vi "Autonomous Independent.vi"() -> ()   [LabVIEW 2016]
doc: "This VI is called when autonomous begins, and will automatically be terminated when autonomous ends. You can carry out timed or sensor driven robot movement independently without needing to return to the caller."
uses:
  <vilib>/Rock Robotics/WPI/Solenoid/WPI_SolenoidValue.ctl
  <vilib>/Rock Robotics/WPI/Utilities/WPI_GetSetVariantRefNum.vi
  <vilib>/Rock Robotics/Network Tables/NT Read String.vi
  <vilib>/Rock Robotics/Network Tables/NT Write Numeric Array.vi
  <vilib>/Rock Robotics/WPI/RobotDrive/WPI_RobotDriveArcadeDrive_Standard(NoSaturation).vi
  <vilib>/Rock Robotics/WPI/Solenoid/WPI_SolenoidSetEnum.vi
panel:
  in  "Reset":bool
  out "Current Movement, for debugging":T1 {"Y Joystick Value" scale=1.0..-1.0; "X Joystick Value" scale=-1.0..1.0}
  in  "Array of robot movements":T2(array[cluster])=[{"X Joystick Value"=0.39393939393939403, "Y Joystick Value"=0.0, "Delay (sec)"=1.0, "Movement Name"="turn"}, {"X Joystick Value"=-0.3737373737373737, "Y Joystick Value"=0.0, "Delay (sec)"=1.0, "Movement Name"="turn back"}] {"Y Joystick Value" scale=1.0..-1.0; "X Joystick Value" scale=-1.0..1.0}
  # "Be sure to right-click and choose Data Operations>>Make Current Value default if you want to save the array values with the VI"
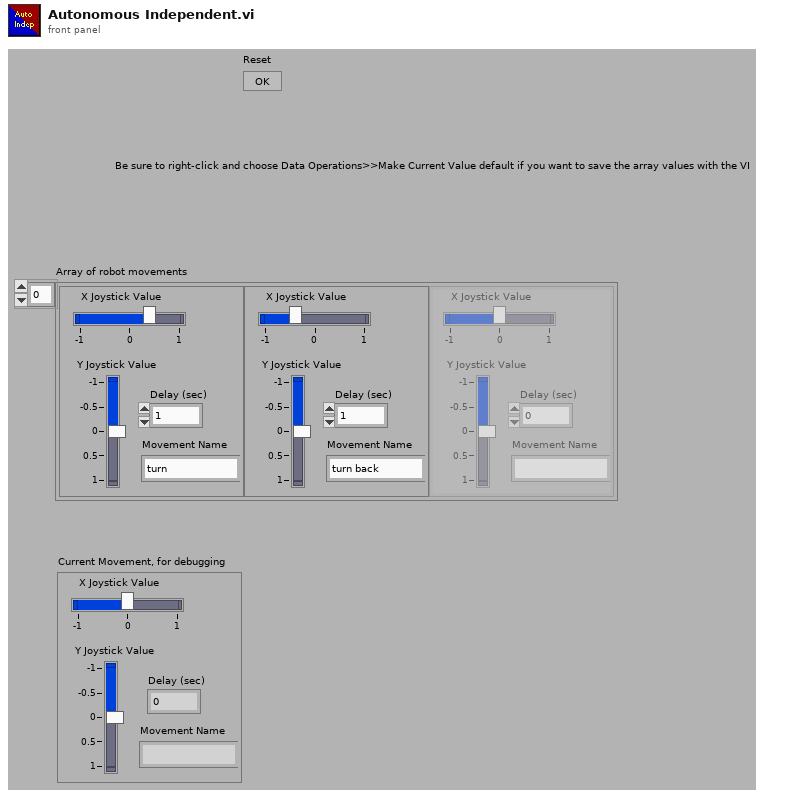
[diagram p1: front panel]
types:
  T1 = cluster{"X Joystick Value":dbl, "Y Joystick Value":dbl, "Delay (sec)":dbl, "Movement Name":string}
  T2 = cluster{"X Joystick Value":dbl, "Y Joystick Value":dbl, "Delay (sec)":dbl, "Movement Name":string}[]
  T3 = typedef "WPI_JoystickDevRef.ctl" = cluster{"Device":T4}
  T4 = typedef "WPI_JoystickDeviceEnum.ctl" = enum16{"USB 0", "USB 1", "USB 2", "USB 3", "USB 4", "USB 5"}
  T5 = typedef "WPI_GyroDevRef.ctl" = cluster{"DevStatus":errorcluster, "Analog Channel":T6, "Offset":dbl, "Gain (VoltsPerDegree/Second)":dbl, "Gyro Type":enum16{"Analog", "XRS450"}, "Handle":i32, "SPI Bus":T7, "Device Found":bool, "Sample Rate":dbl, "Calibrate On Open":bool}
  T6 = typedef "FPGA_AIChannel.ctl" = enum8{"AI 0", "AI 1", "AI 2", "AI 3", "AI MXP 0", "AI MXP 1", "AI MXP 2", "AI MXP 3", "Invalid"}
  T7 = typedef "spi_bus.ctl" = enum16{"SPI On-Board, CS0", "SPI On-Board, CS1", "SPI On-Board, CS2", "SPI On-Board, CS3", "SPI MXP", "Invalid"}
  T8 = typedef "WPI_RobotDriveDevRef.ctl" = cluster{"DevStatus":errorcluster, "Motors[]":T9[], "Square Inputs":bool, "Max Output":dbl}
  T9 = typedef "WPI_MotorControlDeviceRef.ctl" = cluster{"DeviceStatus":errorcluster, "Type":T10, "PWM":cluster{"PWM Channel":T11, "DeadBand":T12}, "CAN":cluster{"Device Number":u8, "SetOutput VI Ref":variant, "GetOutput VI Ref":variant, "Enable VI Ref":variant, "Disable VI Ref":variant, "Data":variant}, "Invert":bool}
  T10 = typedef "WPI_MotorControlType.ctl" = enum16{"PWM", "CAN"}
  T11 = typedef "FPGA_DIOPWMChannel.ctl" = enum8{"PWM 0", "PWM 1", "PWM 2", "PWM 3", "PWM 4", "PWM 5", "PWM 6", "PWM 7", "PWM 8", "PWM 9", "PWM MXP 0", "PWM MXP 1", "PWM MXP 2", "PWM MXP 3", "PWM MXP 4", "PWM MXP 5", "PWM MXP 6", "PWM MXP 7", "PWM MXP 8", "PWM MXP 9", "Invalid"}
  T12 = typedef "WPI_PWMDeadband.ctl" = cluster{"Name":string, "maxPositivePwm":i32, "minPositivePwm":i32, "centerPwm":i32, "maxNegativePwm":i32, "minNegativePwm":i32, "angularRange":u16}
  T13 = typedef "WPI_SolenoidValue.ctl" = enum16{"Off", "On", "Forward", "Reverse"}
  T14 = typedef "WPI_SolenoidDevRef.ctl" = cluster{"DevStatus":errorcluster, "Pneumatics Control Module":u8, "Forward Solenoid Channel":T15, "Reverse Solenoid Channel":T15}
  T15 = typedef "WPI_SolenoidChannel.ctl" = enum8{"Solenoid 0", "Solenoid 1", "Solenoid 2", "Solenoid 3", "Solenoid 4", "Solenoid 5", "Solenoid 6", "Solenoid 7", "Invalid"}
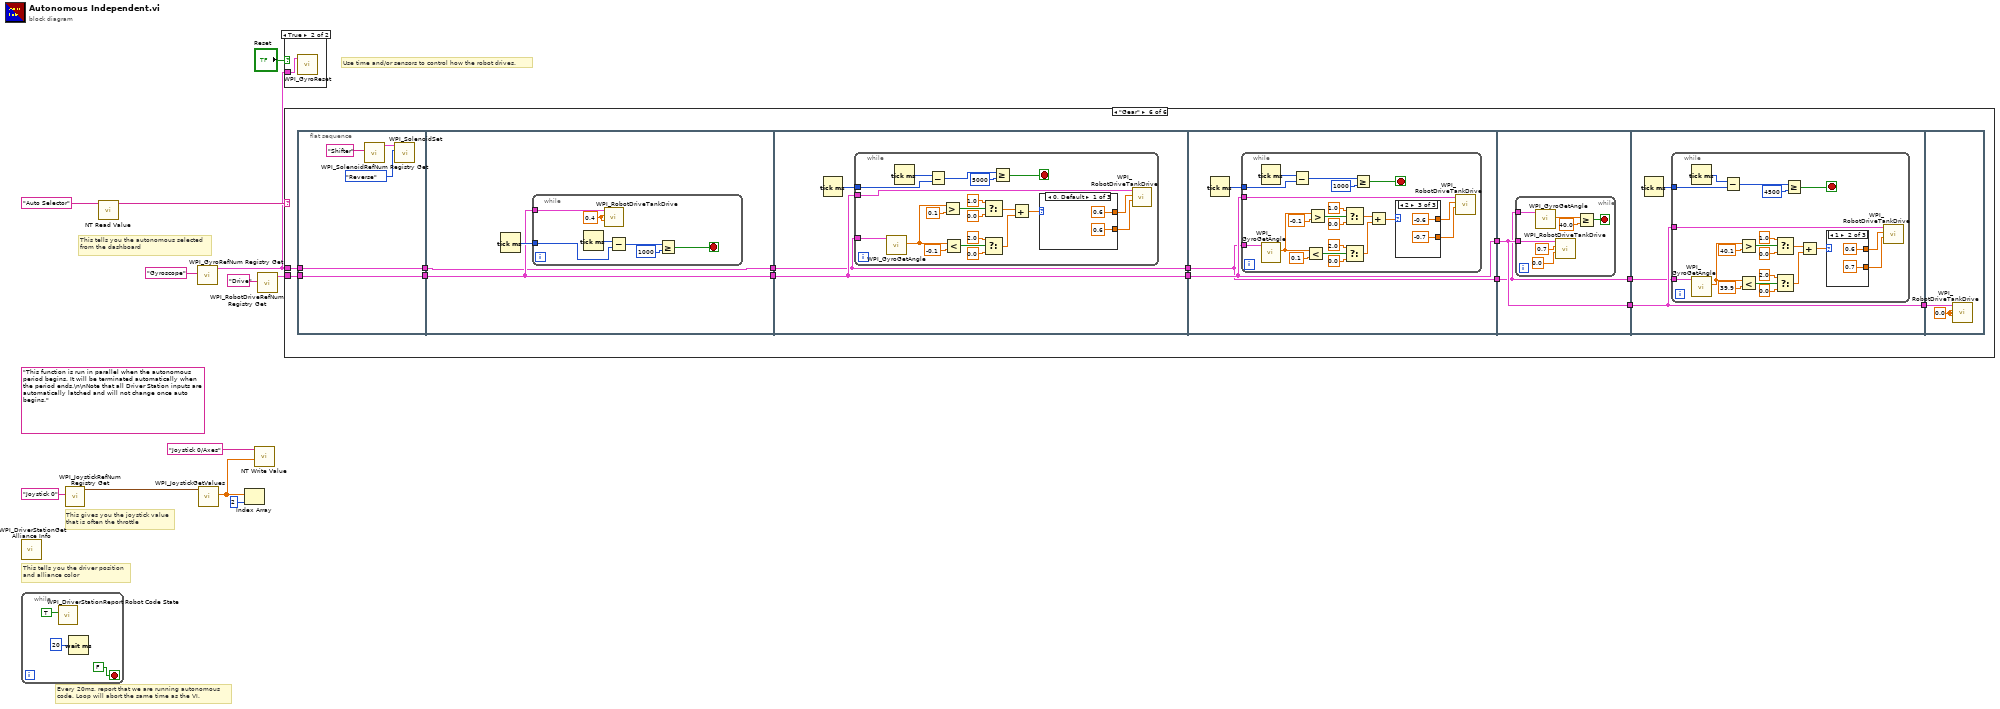
[diagram p0: block diagram]
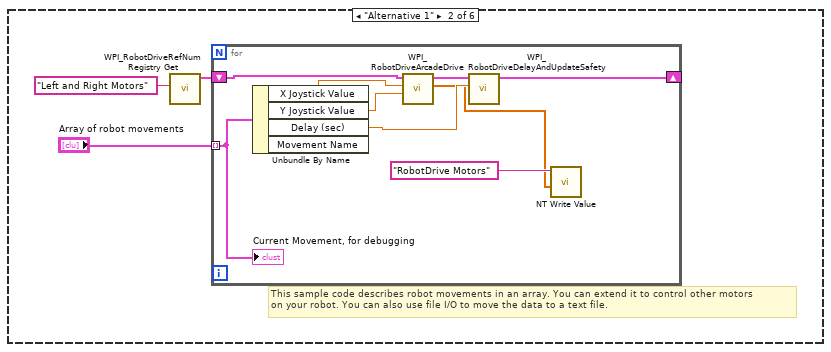
[diagram p4: hidden frame]
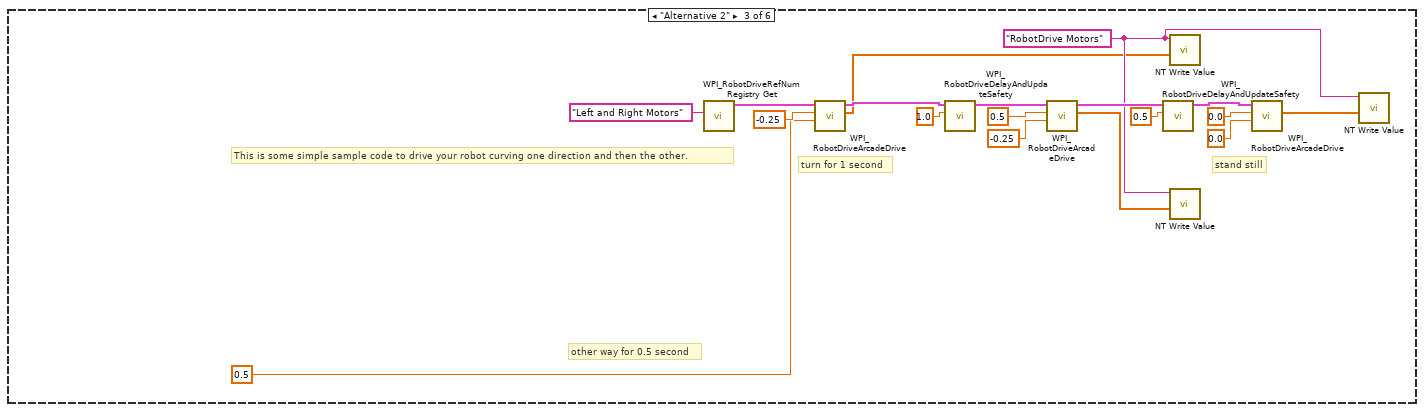
[diagram p5: hidden frame]
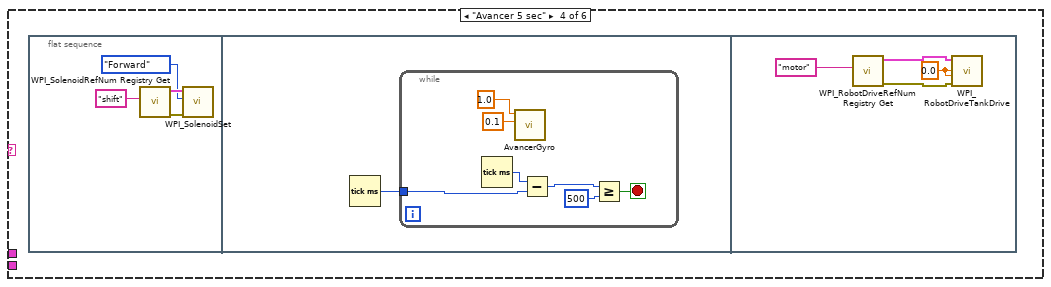
[diagram p6: hidden frame]
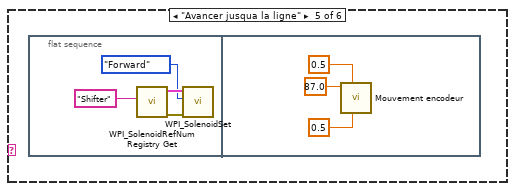
[diagram p7: hidden frame]
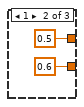
[diagram p8: hidden frame]
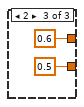
[diagram p9: hidden frame]
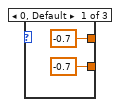
[diagram p10: hidden frame]
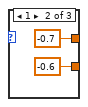
[diagram p11: hidden frame]
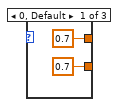
[diagram p12: hidden frame]
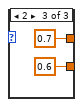
[diagram p13: hidden frame]
diagram:
  (unwired) "This function is run in parallel when the autonomous period begins. It will be terminated automatically when the period ends.\n\nNote that all Driver Station inputs are automatically latched and will not change once auto begins."
  # "This tells you the autonomous selected\nfrom the dashboard"
  # "Every 20ms, report that we are running autonomous\ncode. Loop will abort the same time as the VI."
  # "This gives you the joystick value\nthat is often the throttle"
  # "Use time and/or sensors to control how the robot drives."
  # "This tells you the driver position\nand alliance color"
  n1 = call <vilib>:"WPI_DriverStationGet Alliance Info.vi"() -> ()  [unwired: 12 out]
  n2 = while {
    stop <- FALSE stop-if-true
    n3 = call <vilib>:"WPI_DriverStationReport Robot Code State.vi"("Autonomous"=TRUE) -> ()  [unwired: 10 in, 1 out]
    n4 = Wait (ms)(milliseconds to wait=u32 20) -> ()  [unwired: 1 out]
  }
  n5 = call <vilib>:"WPI_JoystickRefNum Registry Get.vi"("refnum name"="Joystick 0") -> ("JoystickDevRef"=w11:T3)  [unwired: 1 in, 9 out]
  n6 = call-poly <vilib>:"NT Read Value.vi"("Name"="Auto Selector") -> ("String"=w6:string)  [unwired: 9 in, 1 out]
  n7 = call <vilib>:"WPI_GyroRefNum Registry Get.vi"("refnum name"="Gyroscope") -> ("GyroDevRef"=w1:T5)  [unwired: 9 in, 1 out]
  n8 = call <vilib>:"WPI_JoystickGetValues.vi"("JoystickDevRef"=w11) -> ("Axes"=w8:dbl[])  [unwired: 6 in, 4 out]
  n9 = Index Array(array=w8, index=2) -> ()  [unwired: 1 out]
  n10 = call-poly <vilib>:"NT Write Value.vi"("Numeric Array"=w8, "Name"="Joystick 0/Axes") -> ()  [unwired: 9 in, 1 out]
  n11 = call <vilib>:"WPI_RobotDriveRefNum Registry Get.vi"("refnum name"="Drive") -> ("RobotDriveDevRef"=w4:T8)  [unwired: 9 in, 1 out]
  n12 = case shown="True" "Reset" {
    tunnel: w1 -> [_ w16]
    frame False {
    }
    frame True {
      n13 = call <vilib>:"WPI_GyroReset.vi"("GyroDevRef"=w16) -> ()  [unwired: 9 in, 2 out]
    }
  }
  n14 = case shown="\"Gear\"" w6 {
    tunnel: w4 -> [_ _ _ _ _ w82]
    tunnel: w1 -> [_ _ _ _ _ w76]
    frame Default {
      # "You can put your main auto here, or you can right-click on the case and make any\nother frame be the default case."
      # "This is the frame that will execute if no selection is made, or if it is not recognized"
    }
    frame "Alternative 1" {
      # "This sample code describes robot movements in an array. You can extend it to control other motors\non your robot. You can also use file I/O to move the data to a text file."
      n15 = call <vilib>:"WPI_RobotDriveRefNum Registry Get.vi"("refnum name"="Left and Right Motors") -> ("RobotDriveDevRef"=w18:T8)  [unwired: 1 in, 9 out]
      n16 = for {
        shift-right: [w26] -> _
        shift-left: w18 -> [w27]
        tunnel: "Array of robot movements" -> [w22] mode=indexing
        n17 = Unbundle By Name(w22) -> ("X Joystick Value"=w25:dbl, "Y Joystick Value"=w24:dbl, "Delay (sec)"=w23:dbl)  [unwired: 1 out]
        n18 = call-poly <vilib>:"WPI_RobotDriveArcadeDrive.vi"("Y axis value"=w24, "X axis value"=w25, "RobotDriveDevRef"=w27) -> ("Motor Values"=w20:dbl[], "RobotDriveDevRef"=w28:T8)  [unwired: 1 in, 6 out]
        n19 = call <vilib>:"WPI_RobotDriveDelayAndUpdateSafety.vi"("Delay (s)"=w23, "RobotDriveDevRef"=w28) -> ("RobotDriveDevRef 2"=w26:T8)  [unwired: 8 in, 1 out]
        n20 = call-poly <vilib>:"NT Write Value.vi"("Numeric Array"=w20, "Name"="RobotDrive Motors") -> ()  [unwired: 9 in, 1 out]
        "Current Movement, for debugging" <- w22
      }
    }
    frame "Alternative 2" {
      w30 = "RobotDrive Motors" ("Name")
      # "This is some simple sample code to drive your robot curving one direction and then the other."
      # "stand still"
      # "other way for 0.5 second"
      # "turn for 1 second"
      n21 = call <vilib>:"WPI_RobotDriveRefNum Registry Get.vi"("refnum name"="Left and Right Motors") -> ("RobotDriveDevRef"=w46:T8)  [unwired: 1 in, 9 out]
      n22 = call-poly <vilib>:"WPI_RobotDriveArcadeDrive.vi"("Y axis value"=0.5 ("X axis value"), "X axis value"=-0.25, "RobotDriveDevRef"=w46) -> ("Motor Values"=w29:dbl[], "RobotDriveDevRef"=w39:T8)  [unwired: 1 in, 6 out]
      n23 = call <vilib>:"WPI_RobotDriveDelayAndUpdateSafety.vi"("Delay (s)"=1.0, "RobotDriveDevRef"=w39) -> ("RobotDriveDevRef 2"=w40:T8)  [unwired: 8 in, 1 out]
      n24 = call-poly <vilib>:"WPI_RobotDriveArcadeDrive.vi"("Y axis value"=-0.25 ("X axis value"), "X axis value"=0.5, "RobotDriveDevRef"=w40) -> ("Motor Values"=w31:dbl[], "RobotDriveDevRef"=w41:T8)  [unwired: 1 in, 6 out]
      n25 = call <vilib>:"WPI_RobotDriveDelayAndUpdateSafety.vi"("Delay (s)"=0.5, "RobotDriveDevRef"=w41) -> ("RobotDriveDevRef 2"=w42:T8)  [unwired: 8 in, 1 out]
      n26 = call-poly <vilib>:"NT Write Value.vi"("Numeric Array"=w29, "Name"=w30) -> ()  [unwired: 9 in, 1 out]
      n27 = call-poly <vilib>:"NT Write Value.vi"("Numeric Array"=w31, "Name"=w30) -> ()  [unwired: 9 in, 1 out]
      n28 = call-poly <vilib>:"WPI_RobotDriveArcadeDrive.vi"("Y axis value"=0.0 ("X axis value"), "X axis value"=0.0, "RobotDriveDevRef"=w42) -> ("Motor Values"=w32:dbl[])  [unwired: 1 in, 7 out]
      n29 = call-poly <vilib>:"NT Write Value.vi"("Numeric Array"=w32, "Name"=w30) -> ()  [unwired: 9 in, 1 out]
    }
    frame "Avancer 5 sec" {
      n30 = flat-sequence {
        frame #0 {
          n31 = call <vilib>:"WPI_SolenoidRefNum Registry Get.vi"("refnum name"="shift") -> ("error out"=w49:errorcluster, "SolenoidDevRef"=w48:T14)  [unwired: 9 in]
          n32 = call-poly <vilib>:"WPI_SolenoidSet.vi"("error in (no error)"=w49, "Value"=WPI_SolenoidValue."Forward", "SolenoidDevRef"=w48) -> ()  [unwired: 7 in, 2 out]
        }
        frame #1 {
          n33 = Tick Count (ms)() -> (millisecond timer value=w51:u32)
          n34 = while {
            tunnel: w51 -> [w55]
            stop <- w52 stop-if-true
            n35 = Tick Count (ms)() -> (millisecond timer value=w56:u32)
            n36 = call "AvancerGyro.vi"("Ajustement"=0.1, "Vitesse"=1.0) -> ()  [unwired: 10 in]
            n37 = Subtract(x=w56, y=w55) -> (x-y=w54:u32)
            n38 = Greater Or Equal?(x=w54, y=u32 500) -> (x >= y?=w52:bool)
          }
        }
        frame #2 {
          w62 = 0.0 ("Left axis value")
          n39 = call <vilib>:"WPI_RobotDriveRefNum Registry Get.vi"("refnum name"="motor") -> ("error out"=w61:errorcluster, "RobotDriveDevRef"=w60:T8)  [unwired: 9 in]
          n40 = call <vilib>:"WPI_RobotDriveTankDrive.vi"("error in (no error)"=w61, "Right axis value"=w62, "Left axis value"=w62, "RobotDriveDevRef"=w60) -> ()  [unwired: 5 in, 3 out]
        }
      }
    }
    frame "Avancer jusqua la ligne" {
      n41 = flat-sequence {
        frame #0 {
          n42 = call <vilib>:"WPI_SolenoidRefNum Registry Get.vi"("refnum name"="Shifter") -> ("error out"=w65:errorcluster, "SolenoidDevRef"=w64:T14)  [unwired: 9 in]
          n43 = call-poly <vilib>:"WPI_SolenoidSet.vi"("error in (no error)"=w65, "Value"=WPI_SolenoidValue."Forward", "SolenoidDevRef"=w64) -> ()  [unwired: 7 in, 2 out]
        }
        frame #1 {
          n44 = call "Mouvement encodeur.vi"("Vitesse initiale"=0.5, "Temps acceleration"=0.5, "Distance"=87.0) -> ()  [unwired: 9 in]
        }
      }
    }
    frame "Gear" {
      n45 = flat-sequence {
        tunnel: [w84] -> w80
        tunnel: w82 -> [w84]
        tunnel: [w83] -> w77
        tunnel: w76 -> [w83]
        tunnel: w80 -> [w89]
        tunnel: [w89] -> w79
        tunnel: [w88] -> w78
        tunnel: w77 -> [w88]
        tunnel: w79 -> [w100]
        tunnel: [w100] -> w81
        tunnel: w78 -> [w98]
        tunnel: [w98] -> w74
        tunnel: w81 -> [w129]
        tunnel: [w129] -> w75
        tunnel: w74 -> [w128]
        tunnel: [w128] -> w73
        tunnel: w75 -> [w159]
        tunnel: [w159] -> w72
        tunnel: w73 -> [w158]
        tunnel: [w158] -> w70
        tunnel: w72 -> [w168]
        tunnel: [w168] -> w71
        tunnel: w70 -> [w167]
        tunnel: w71 -> [w197]
        frame #0 {
          n46 = call <vilib>:"WPI_SolenoidRefNum Registry Get.vi"("refnum name"="Shifter") -> ("SolenoidDevRef"=w87:T14)  [unwired: 9 in, 1 out]
          n47 = call-poly <vilib>:"WPI_SolenoidSet.vi"("Value"=WPI_SolenoidValue."Reverse", "SolenoidDevRef"=w87) -> ()  [unwired: 8 in, 2 out]
        }
        frame #1 {
          n48 = Tick Count (ms)() -> (millisecond timer value=w90:u32)
          n49 = while {
            tunnel: w89 -> [w96]
            tunnel: w90 -> [w94]
            stop <- w91 stop-if-true
            w97 = 0.4 ("Left axis value")
            n50 = Tick Count (ms)() -> (millisecond timer value=w95:u32)
            n51 = call <vilib>:"WPI_RobotDriveTankDrive.vi"("Right axis value"=w97, "Left axis value"=w97, "RobotDriveDevRef"=w96) -> ()  [unwired: 6 in, 3 out]
            n52 = Subtract(x=w95, y=w94) -> (x-y=w93:u32)
            n53 = Greater Or Equal?(x=w93, y=u32 1000) -> (x >= y?=w91:bool)
          }
        }
        frame #2 {
          n54 = Tick Count (ms)() -> (millisecond timer value=w99:u32)
          n55 = while {
            tunnel: w100 -> [w121]
            tunnel: w99 -> [w119]
            tunnel: w98 -> [w115]
            stop <- w116 stop-if-true
            n56 = call <vilib>:"WPI_GyroGetAngle.vi"("GyroDevRef"=w115) -> ("Angle"=w102:dbl)  [unwired: 6 in, 4 out]
            n57 = Tick Count (ms)() -> (millisecond timer value=w120:u32)
            n58 = Subtract(x=w120, y=w119) -> (x-y=w118:u32)
            n59 = Greater?(x=w102, y=0.1) -> (0:w113:bool)
            n60 = Less?(x=w102, y=-0.1) -> (x < y?=w101:bool)
            n61 = Select(t=1.0, s=w113, f=0.0) -> (s? t:f=w108:dbl)
            n62 = Select(t=2.0, s=w101, f=0.0) -> (s? t:f=w107:dbl)
            n63 = Greater Or Equal?(x=w118, y=u32 5000) -> (x >= y?=w116:bool)
            n64 = Add(x=w108, y=w107) -> (x+y=w106:dbl)
            n65 = case shown="0, Default" w106 {
              tunnel: [0.6 ("t") 0.5 ("t") 0.6 ("t")] -> w105
              tunnel: [0.6 ("f") 0.6 ("f") 0.5 ("f")] -> w104
              frame 0, Default {
              }
              frame 1 {
              }
              frame 2 {
              }
            }
            n66 = call <vilib>:"WPI_RobotDriveTankDrive.vi"("Right axis value"=w104, "Left axis value"=w105, "RobotDriveDevRef"=w121) -> ()  [unwired: 6 in, 3 out]
          }
        }
        frame #3 {
          n67 = Tick Count (ms)() -> (millisecond timer value=w130:u32)
          n68 = while {
            tunnel: w129 -> [w134]
            tunnel: w130 -> [w150]
            tunnel: w128 -> [w131]
            stop <- w147 stop-if-true
            n69 = Tick Count (ms)() -> (millisecond timer value=w151:u32)
            n70 = call <vilib>:"WPI_GyroGetAngle.vi"("GyroDevRef"=w131) -> ("Angle"=w145:dbl)  [unwired: 6 in, 4 out]
            n71 = Subtract(x=w151, y=w150) -> (x-y=w149:u32)
            n72 = Less?(x=w145, y=0.1) -> (x < y?=w146:bool)
            n73 = Greater?(x=w145, y=-0.1) -> (0:w136:bool)
            n74 = Select(t=1.0, s=w136, f=0.0) -> (s? t:f=w141:dbl)
            n75 = Select(t=2.0, s=w146, f=0.0) -> (s? t:f=w142:dbl)
            n76 = Greater Or Equal?(x=w149, y=u32 1000) -> (x >= y?=w147:bool)
            n77 = Add(x=w141, y=w142) -> (x+y=w143:dbl)
            n78 = case shown="2" w143 {
              tunnel: [-0.7 ("t") -0.7 ("t") -0.6 ("t")] -> w133
              tunnel: [-0.7 ("f") -0.6 ("f") -0.7 ("f")] -> w132
              frame 0, Default {
              }
              frame 1 {
              }
              frame 2 {
              }
            }
            n79 = call <vilib>:"WPI_RobotDriveTankDrive.vi"("Right axis value"=w132, "Left axis value"=w133, "RobotDriveDevRef"=w134) -> ()  [unwired: 6 in, 3 out]
          }
        }
        frame #4 {
          n80 = while {
            tunnel: w158 -> [w163]
            tunnel: w159 -> [w160]
            stop <- w164 stop-if-true
            n81 = call <vilib>:"WPI_GyroGetAngle.vi"("GyroDevRef"=w163) -> ("Angle"=w166:dbl)  [unwired: 6 in, 4 out]
            n82 = call <vilib>:"WPI_RobotDriveTankDrive.vi"("Right axis value"=0.0, "Left axis value"=0.7, "RobotDriveDevRef"=w160) -> ()  [unwired: 6 in, 3 out]
            n83 = Greater Or Equal?(x=w166, y=40.0) -> (x >= y?=w164:bool)
          }
        }
        frame #5 {
          n84 = Tick Count (ms)() -> (millisecond timer value=w169:u32)
          n85 = while {
            tunnel: w168 -> [w190]
            tunnel: w169 -> [w188]
            tunnel: w167 -> [w184]
            stop <- w185 stop-if-true
            n86 = Tick Count (ms)() -> (millisecond timer value=w189:u32)
            n87 = call <vilib>:"WPI_GyroGetAngle.vi"("GyroDevRef"=w184) -> ("Angle"=w171:dbl)  [unwired: 6 in, 4 out]
            n88 = Subtract(x=w189, y=w188) -> (x-y=w187:u32)
            n89 = Greater?(x=w171, y=40.1) -> (0:w182:bool)
            n90 = Less?(x=w171, y=39.9) -> (x < y?=w170:bool)
            n91 = Select(t=1.0, s=w182, f=0.0) -> (s? t:f=w177:dbl)
            n92 = Select(t=2.0, s=w170, f=0.0) -> (s? t:f=w176:dbl)
            n93 = Greater Or Equal?(x=w187, y=u32 4500) -> (x >= y?=w185:bool)
            n94 = Add(x=w177, y=w176) -> (x+y=w175:dbl)
            n95 = case shown="1" w175 {
              tunnel: [0.7 ("t") 0.6 ("t") 0.7 ("t")] -> w174
              tunnel: [0.7 ("f") 0.7 ("f") 0.6 ("f")] -> w173
              frame 0, Default {
              }
              frame 1 {
              }
              frame 2 {
              }
            }
            n96 = call <vilib>:"WPI_RobotDriveTankDrive.vi"("Right axis value"=w173, "Left axis value"=w174, "RobotDriveDevRef"=w190) -> ()  [unwired: 6 in, 3 out]
          }
        }
        frame #6 {
          w198 = 0.0 ("Left axis value")
          n97 = call <vilib>:"WPI_RobotDriveTankDrive.vi"("Right axis value"=w198, "Left axis value"=w198, "RobotDriveDevRef"=w197) -> ()  [unwired: 6 in, 3 out]
        }
      }
    }
  }
